vi "Set Attributes.vi"(8 "error in (no error)":errorcluster, 11 "Conditional Dialog in":refnum<class "Conditional Dialog.lvclass">) -> (0 "error out":errorcluster, 3 "Conditional Dialog out":refnum<class "Conditional Dialog.lvclass">)   [LabVIEW 2017, in "Conditional Dialog.lvclass"]
uses:
  Conditional Dialog.lvclass
  ITest Executive Builder Dialog/ITest Executive Builder Dialog.lvclass
  <vilib>/gpm_packages/@cs/test-executive/Source/Test Executive/TestExecutive Ref/TestExecutive Ref.lvclass
  5f769910-1e0f-4ec2-846f-ffdb4f9bf496.vi
  9047d4da-06b1-4e6c-8248-6ac24da04460.vi
  71333869-f5de-41ab-b41d-cf8ee9c94312.vi
  c0337e01-bd89-4521-aed9-e3b53a67ddf9.vi
  C:/Users/jonmc/Documents/Git/Test Executive Builder/Source/Test Executive Builder Dialogs/ITest Executive Builder Dialog/ITest Executive Builder Dialog.lvclass
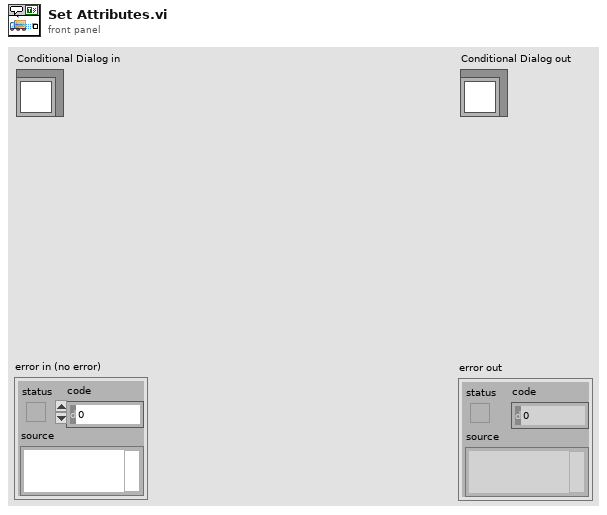
[diagram p1: front panel]
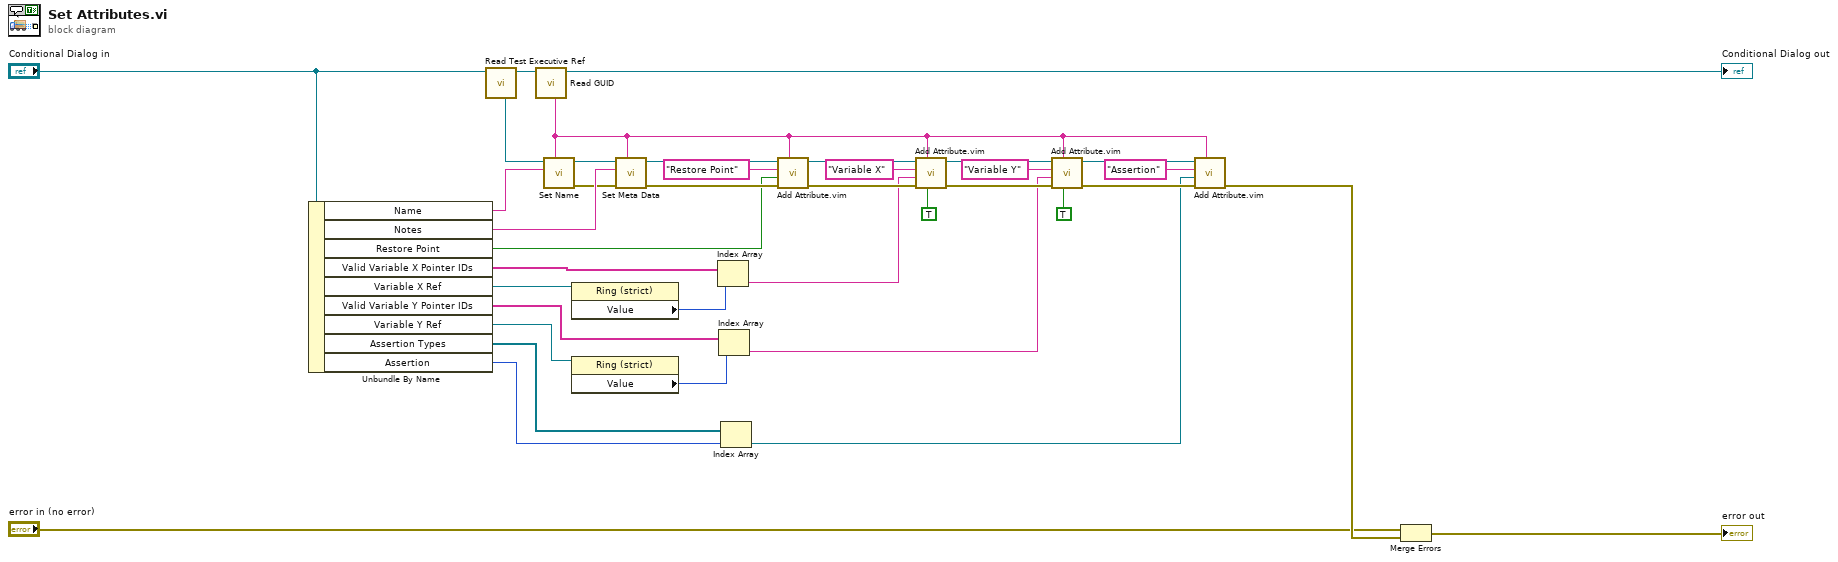
[diagram p0: block diagram]
diagram:
  n1 = Unbundle By Name("Conditional Dialog in") -> ("Name"=w36:string, "Notes"=w34:string, "Restore Point"=w29:bool, "Valid Variable X Pointer IDs"=w26:string[], "Variable X Ref"=w28:refnum<vi>, "Valid Variable Y Pointer IDs"=w24:string[], "Variable Y Ref"=w27:refnum<vi>, "Assertion Types"=w8:refnum<class "Assert.lvclass">[], "Assertion"=w7:u16)
  n2 = call "Read Test Executive Ref.vi"("ITest Executive Builder Dialog in"="Conditional Dialog in") -> ("ITest Executive Builder Dialog out"=w38:refnum<class "Conditional Dialog.lvclass">, "Test Executive Ref"=w37:refnum<data-value>)  [unwired: 9 in]
  n3 = call "Read GUID.vi"("ITest Executive Builder Dialog in"=w38) -> ("ITest Executive Builder Dialog out"=→"Conditional Dialog out":refnum<class "Conditional Dialog.lvclass">, "GUID"=w5:string)  [unwired: 9 in]
  n4 = call <vilib>:"Set Name.vi"("Unique ID"=w5, "Name"=w36, "Test Executive Ref"=w37) -> ("error out"=w33:errorcluster, "Test Executive Ref out"=w35:refnum<data-value>)  [unwired: 7 in]
  n5 = property class="Ring (strict)"(reference=w28) -> ("Value"=w25:u16)  [unwired: 1 in, 2 out]
  n6 = property class="Ring (strict)"(reference=w27) -> ("Value"=w23:u16)  [unwired: 1 in, 2 out]
  n7 = call <vilib>:"Set Meta Data.vi"("Unique ID"=w5, "error in (no error)"=w33, "Meta Data"=w34, "Test Executive Ref"=w35) -> ("error out"=w30:errorcluster, "Test Executive Ref out"=w31:refnum<data-value>)  [unwired: 6 in]
  n8 = Index Array(array=w26, index=w25) -> (element=w14:string)
  n9 = Index Array(array=w24, index=w23) -> (element=w13:string)
  n10 = Index Array(array=w8, index=w7) -> (element=w6:refnum<class "Assert.lvclass">)
  n11 = call "Add Attribute.vim"("ID"=w5, "error in (no error)"=w30, "Attribute"=w29, "Attribute Name"="Restore Point", "Test Executive Ref"=w31) -> ("error out"=w19:errorcluster, "Test Executive Ref out"=w22:refnum<data-value>)  [unwired: 3 in, 2 out]
  n12 = call "Add Attribute.vim"("Pointer?"=TRUE, "ID"=w5, "error in (no error)"=w19, "Attribute"=w14, "Attribute Name"="Variable X", "Test Executive Ref"=w22) -> ("error out"=w20:errorcluster, "Test Executive Ref out"=w21:refnum<data-value>)  [unwired: 2 in, 2 out]
  n13 = call "Add Attribute.vim"("Pointer?"=TRUE, "ID"=w5, "error in (no error)"=w20, "Attribute"=w13, "Attribute Name"="Variable Y", "Test Executive Ref"=w21) -> ("error out"=w12:errorcluster, "Test Executive Ref out"=w10:refnum<data-value>)  [unwired: 2 in, 2 out]
  n14 = call "Add Attribute.vim"("ID"=w5, "error in (no error)"=w12, "Attribute"=w6, "Attribute Name"="Assertion", "Test Executive Ref"=w10) -> ("error out"=w11:errorcluster)  [unwired: 3 in, 3 out]
  n15 = Merge Errors("error in (no error)", w11) -> (→"error out":errorcluster)
